vi "Encoder_Read_sub_VI.vi"() -> ()   [LabVIEW 2017]
uses:
  <vilib>/myRIO/Common/Instrument Driver Framework/myRIO v1.0/Encoder/typedefs/Encoder Signal Mode.ctl
  <vilib>/myRIO/Instrument Drivers/Onboard IO/Encoder/typedefs/Encoder Reference.ctl
  <vilib>/myRIO/Common/Instrument Driver Framework/Utilities/typedefs/myRIO Generic Hardware Reference.ctl
  <vilib>/myRIO/Common/Instrument Driver Framework/Utilities/typedefs/Hardware Version Enum.ctl
  <vilib>/myRIO/Common/Instrument Driver Framework/Utilities/typedefs/myRIO v1.0 Reference.ctl
  <vilib>/myRIO/Common/Instrument Driver Framework/Utilities/typedefs/Generic FPGA Reference.ctl
  <vilib>/myRIO/Common/Instrument Driver Framework/myRIO v1.0/Encoder/typedefs/Encoder Channels Enum.ctl
  <vilib>/myRIO/Common/Instrument Driver Framework/myRIO v1.0/Encoder/typedefs/Encoder Configuration v1.0.ctl
  <vilib>/userdefined/High Color/nirio_resource_hc.ctl
  <vilib>/myRIO/Common/Instrument Driver Framework/Utilities/vis/Is FPGA Ref Available.vi
  <vilib>/myRIO/Common/Instrument Driver Framework/myRIO v1.0/Encoder/vis/myRIO v1.1 Open Encoder.vi
  <vilib>/myRIO/Instrument Drivers/Onboard IO/Encoder/vis/Read.vi
  <vilib>/myRIO/Common/Instrument Driver Framework/Utilities/vis/Validate Channels.vi
  <vilib>/myRIO/Common/Instrument Driver Framework/myRIO v1.0/Encoder/vis/myRIO v1.0 Reserve Encoder.vi
  <vilib>/myRIO/Common/Instrument Driver Framework/myRIO v1.0/Encoder/vis/myRIO v1.0 Build MUX Configuration Encoder.vi
  <vilib>/myRIO/Common/Instrument Driver Framework/myRIO v1.0/Resource Manager/vis/myRIO v1.0 Reserve Channel List.vi
  <vilib>/myRIO/Common/Instrument Driver Framework/myRIO v1.0/Resource Manager/vis/myRIO v1.0 Create Configuration List.vi
  <vilib>/myRIO/Common/Instrument Driver Framework/myRIO v1.0/Resource Manager/vis/myRIO v1.0 Reserve Channel.vi
  <vilib>/myRIO/Common/Instrument Driver Framework/myRIO v1.0/Resource Manager/vis/myRIO v1.0 Unreserve Channel.vi
  <vilib>/myRIO/Common/Instrument Driver Framework/myRIO v1.0/Resource Manager/vis/myRIO v1.0 Build Mutex Name.vi
  <vilib>/Utility/VariantDataType/GetNumericInfo.vi
  <vilib>/Utility/error.llb/Error Cluster From Error Code.vi
  <vilib>/myRIO/Common/Instrument Driver Framework/myRIO v1.0/myRIO v1.1 Open.vi
  <vilib>/myRIO/Common/Instrument Driver Framework/Utilities/vis/IO Manager.vi
  <vilib>/myRIO/Common/Instrument Driver Framework/Utilities/vis/Configuration Manager.vi
  <vilib>/myRIO/Common/Instrument Driver Framework/myRIO v1.0/Resource Manager/vis/myRIO v1.0 Configure IO.vi
  <vilib>/myRIO/Common/Instrument Driver Framework/myRIO v1.0/myRIO v1.0 Close.vi
  <vilib>/myRIO/Common/Instrument Driver Framework/myRIO v1.0/Encoder/vis/myRIO v1.0 Configure Encoder.vi
  <vilib>/myRIO/Common/Instrument Driver Framework/myRIO v1.0/Encoder/vis/myRIO v1.0 Read Encoder.vi
  <vilib>/myRIO/Express VI/Onboard IO/Encoder/Encoder Express VI.xnode
  <vilib>/myRIO/Common/Instrument Driver Framework/myRIO v1.0/Encoder/typedefs/Encoder Count Direction Enum.ctl
  <vilib>/myRIO/Instrument Drivers/Onboard IO/Encoder/vis/myRIO Encoder Open.xnode
  <vilib>/myRIO/Instrument Drivers/Onboard IO/Encoder/Encoder.lvlib
panel:
  out "X-axis direction":enum16{"Counting Up", "Counting Down"}(ring)
  out "Y-axis direction":enum16{"Counting Up", "Counting Down"}(ring)
  out "Encoder Output":T1
  in  "Encoder Input":T1
  out "error out":errorcluster
  in  "error in (no error)":errorcluster
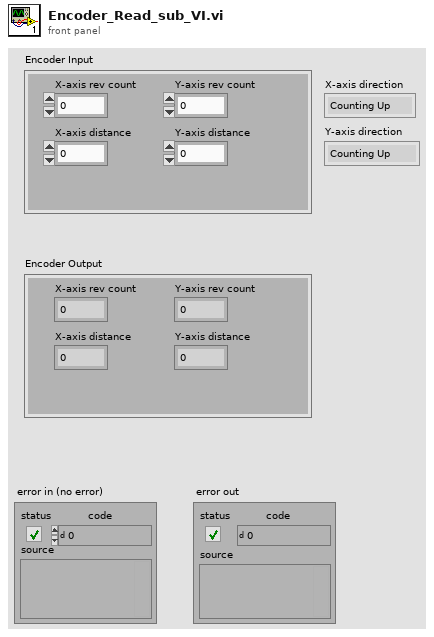
[diagram p1: front panel]
types:
  T1 = cluster{"Y-axis rev count":dbl, "Y-axis distance":dbl, "X-axis rev count":dbl, "X-axis distance":dbl}
  T2 = typedef "Encoder Count Direction Enum.ctl" = enum16{"Counting Up", "Counting Down"}
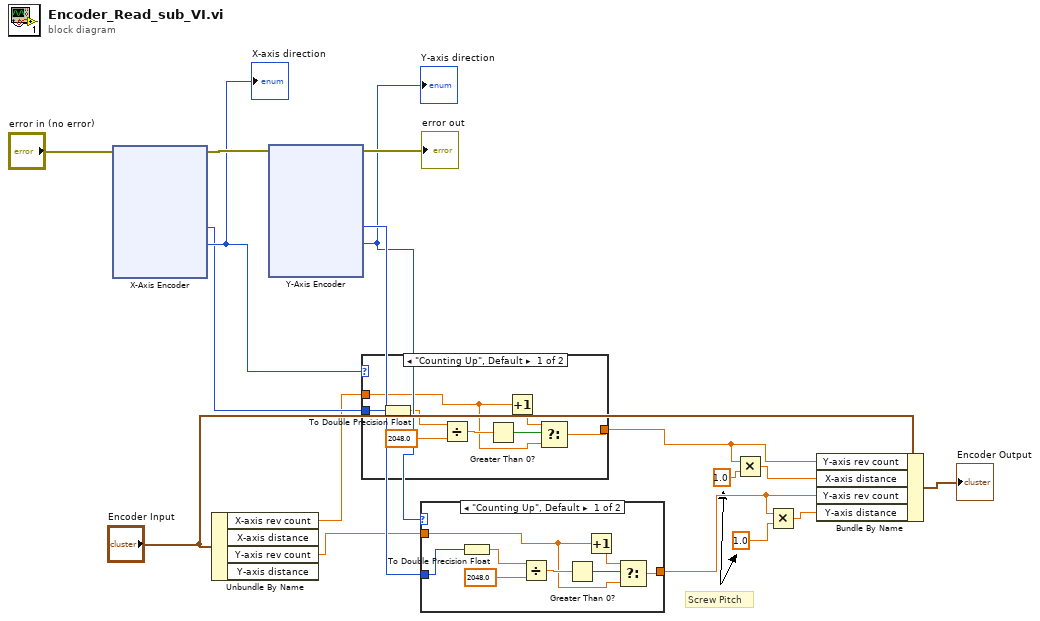
[diagram p0: block diagram]
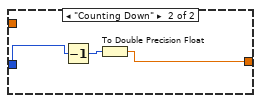
[diagram p2: hidden frame]
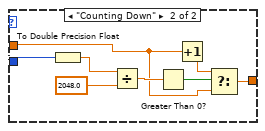
[diagram p3: hidden frame]
diagram:
  # "Screw Pitch"
  n1 = xnode "X-Axis Encoder"("error in (no error)"="error in (no error)") -> ("Counter Value"=w10:i32, "Counter Direction"=w11:T2, "error out"=w14:errorcluster)  [unwired: 1 in, 1 out]
  "X-axis direction" <- w11
  n2 = Unbundle By Name("Encoder Input") -> ("X-axis rev count"=w8:dbl, "Y-axis rev count"=w7:dbl)  [unwired: 2 out]
  n3 = xnode "Y-Axis Encoder"("error in (no error)"=w14) -> ("Counter Value"=w12:i32, "Counter Direction"=w9:enum16{"Counting Up", "Counting Down"}, "error out"=→"error out":errorcluster)  [unwired: 1 in, 1 out]
  "Y-axis direction" <- w9
  n4 = case shown="\"Counting Up\", Default" w11 {
    tunnel: w10 -> [w25 w27]
    tunnel: [w18 w26] -> w1
    tunnel: w8 -> [w19 w28]
    frame "Counting Up", Default {
      n5 = To Double Precision Float(number=w25) -> (double precision float=w21:dbl)
      n6 = Divide(x=w21, y=2048.0) -> (x/y=w23:dbl)
      n7 = Greater Than 0?(x=w23) -> (x > 0?=w24:bool)
      n8 = Increment(x=w19) -> (x+1=w20:dbl)
      n9 = Select(t=w20, s=w24, f=w19) -> (s? t:f=w18:dbl)
    }
    frame "Counting Down" {
      n10 = To Double Precision Float(number=w27) -> (double precision float=w30:dbl)
      n11 = Divide(x=w30, y=2048.0) -> (x/y=w32:dbl)
      n12 = Greater Than 0?(x=w32) -> (x > 0?=w33:bool)
      n13 = Increment(x=w28) -> (x+1=w29:dbl)
      n14 = Select(t=w29, s=w33, f=w28) -> (s? t:f=w26:dbl)
    }
  }
  n15 = case shown="\"Counting Up\", Default" w9 {
    tunnel: w12 -> [w36 w42]
    tunnel: [w34 w44] -> w6
    tunnel: w7 -> [w35 _]
    frame "Counting Up", Default {
      n16 = To Double Precision Float(number=w36) -> (double precision float=w38:dbl)
      n17 = Divide(x=w38, y=2048.0) -> (x/y=w40:dbl)
      n18 = Greater Than 0?(x=w40) -> (x > 0?=w41:bool)
      n19 = Increment(x=w35) -> (x+1=w37:dbl)
      n20 = Select(t=w37, s=w41, f=w35) -> (s? t:f=w34:dbl)
    }
    frame "Counting Down" {
      n21 = Decrement(x=w42) -> (x-1=w43:i32)
      n22 = To Double Precision Float(number=w43) -> (double precision float=w44:dbl)
    }
  }
  n23 = Multiply(x=w1, y=1.0) -> (x*y=w2:dbl)
  n24 = Multiply(x=w6, y=1.0) -> (x*y=w3:dbl)
  n25 = Bundle By Name(cluster="Encoder Input", "Y-axis rev count"=w1, "X-axis distance"=w2, "Y-axis rev count"=w6, "Y-axis distance"=w3) -> (→"Encoder Output":T1)
